vi "Add_Extra_Command.vi"(1 "Traverse line":T1 {"Row Duration (mins)" format="%#.1f"; "Row No" min=0; "Trace Gas Concentration (%)" min=0.0 format="%#.2f"; "Emission Rate (l/min)" format="%#.2f"; "Tunnel Speed" format="%#.2f"; "Start X" format="%#.2f"; "Start Y" format="%#.2f"; "Start Z" format="%#.2f"; "End X" format="%#.2f"; "End Y" format="%#.2f"; "End Z" format="%#.2f"; "Averaging time (min)" min=0.0 format="%#.2f"}, 2 "Extra Command":string) -> (0 "Traverse line Out":T1 {"Row Duration (mins)" format="%#.1f"; "Row No" min=0; "Trace Gas Concentration (%)" min=0.0 format="%#.2f"; "Emission Rate (l/min)" format="%#.2f"; "Tunnel Speed" format="%#.2f"; "Start X" format="%#.2f"; "Start Y" format="%#.2f"; "Start Z" format="%#.2f"; "End X" format="%#.2f"; "End Y" format="%#.2f"; "End Z" format="%#.2f"; "Averaging time (min)" min=0.0 format="%#.2f"})   [LabVIEW 2010]
uses:
  Gen Trav/Traverse_cluster.ctl
  Gen Trav/Spacing.ctl
  Controls/Multi_run_mode.ctl
panel:
  # "X           Y            Z"
  # "Start"
  # "End"
  # "X           Y            Z"
  # "Start"
  # "End"
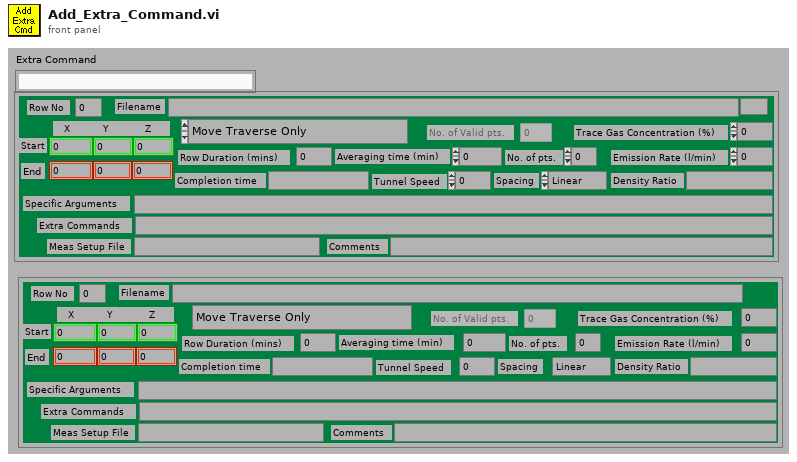
[diagram p1: front panel]
types:
  T1 = typedef "Traverse_cluster.ctl" = cluster{"Start X":dbl, "Start Y":dbl, "Start Z":dbl, "End X":dbl, "End Y":dbl, "End Z":dbl, "No. of pts.":i32, "Spacing":T2, "Filename":path, "Tunnel Speed":dbl, "Averaging time (min)":dbl, "Extra Commands":string, "Specific Arguments":string, "Emission Rate (l/min)":dbl, "Trace Gas Concentration (%)":dbl, "Density Ratio":string, "Comments":string, "Row No":i32, "Row Type Selector":T3, "Completion time":string, "Row Duration (mins)":dbl, "No. of Valid pts.":i32, "Meas Setup File":string}
  T2 = typedef "Spacing.ctl" = enum16{"Linear", "Log", "Gauss", "Specified", "N/A"}
  T3 = typedef "Multi_run_mode.ctl" = enum16{"Move Traverse Only", "Set Tunnel Speed Only", "Set Source Only", "Set Measurement Conditions", "Single Measurement", "Vertical Profile", "Lateral Profile", "Longitudinal Profile", "Explore Volume", "Multi-Axis Profile", "Auto Calibrate", "Meas Fast FID Bkgnd", "Check Beam Power", "Scanning Valve Measurement", "Run VI Named:", "Set ADAM Ch", "Wait (minutes)", "Send Message", "Synchronize With:", "Fall Back to this Row", "Turn Off Row Repeating", "Blank Row"}
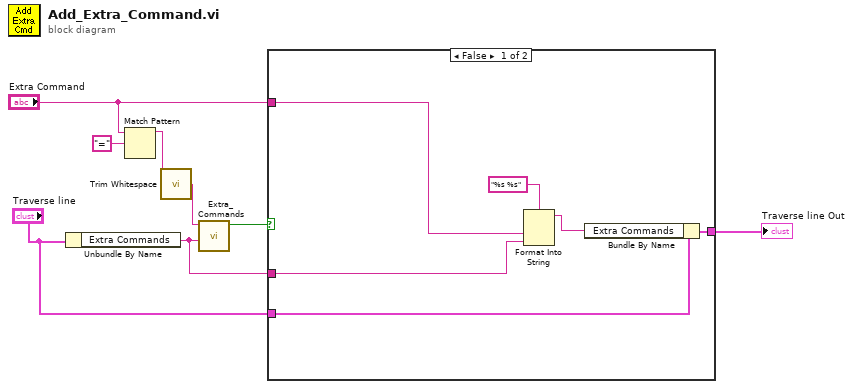
[diagram p0: block diagram]
diagram:
  n1 = Unbundle By Name("Traverse line") -> ("Extra Commands"=w3:string)
  n2 = Match Pattern(string="Extra Command", regular expression="=") -> (before substring=w7:string)  [unwired: 4 out]
  n3 = call <vilib>:"Trim Whitespace.vi"("string"=w7) -> ("trimmed string"=w1:string)  [unwired: 1 in]
  n4 = call "Extra_Commands.vi"("String to Search"=w3, "Command"=w1) -> ("Command Found"=w6:bool)  [unwired: 1 in, 4 out]
  n5 = case shown="False" w6 {
    tunnel: [w13 w15] -> w5
    tunnel: "Traverse line" -> [w14 w15]
    tunnel: w3 -> [w12 _]
    tunnel: "Extra Command" -> [w11 _]
    frame False {
      n6 = Format Into String(format string="%s %s", w11, w12) -> (resulting string=w10:string)  [unwired: 2 in, 1 out]
      n7 = Bundle By Name(cluster=w14, "Extra Commands"=w10) -> (w13:T1)
    }
    frame True {
    }
  }
  "Traverse line Out" <- w5
